vi "Complex Characteristic Polynomial.vi"(3 "Input Matrix":T1) -> (0 "error":i32, 1 "Characteristic Polynomial":cdb[](array[numeric]))   [LabVIEW 2017, in "NI_AALPro.lvlib"]
doc: "Computes the characteristic polynomial of <B>Input Matrix</B>. Wire data to the <B>Input Matrix</B> input to determine the polymorphic instance to use or manually select the instance."
uses:
  NI_AALPro.lvlib
  ComplexMatrix.ctl
  <resource>/lvanlys.dll
  NI_Matrix.lvlib
panel:
  # "Complex Matrix Characteristic Polynomial"
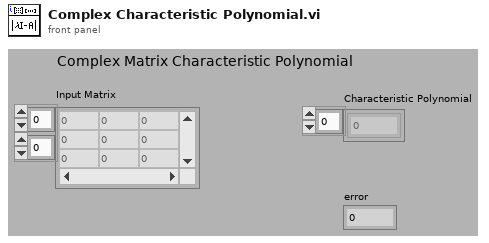
[diagram p1: front panel]
types:
  T1 = typedef "NI_Matrix.lvlib/ComplexMatrix.ctl" = cdb[][]
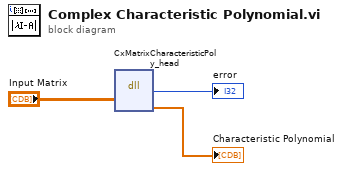
[diagram p0: block diagram]
diagram:
  n1 = dll-call lib="C:/Program Files (x86)/National Instruments/LabVIEW 2017/resource/lvanlys.*" fn="CxMatrixCharacteristicPoly_head"("aH"="Input Matrix") -> ("return type"=→"error":i32, "Characteristic Polynomial"=→"Characteristic Polynomial":cdb[])  [unwired: 4 in, 3 out]
